vi "Initialise 3 cameras.vi"() -> (0 "Error Out":errorcluster, 1 "Blue camera ref":refnum<k24>, 2 "Green camera ref":refnum<k24>, 3 "Red camera ref":refnum<k24>)   [LabVIEW 2017]
uses:
  C:/Program Files/National Instruments/LabVIEW 2017/instr.lib/IDS/ueye.NET/uEyeDotNet.dll
panel:
  out "Serial Number 3":string
  out "Serial Number 2":string
  out "Serial Number 1":string
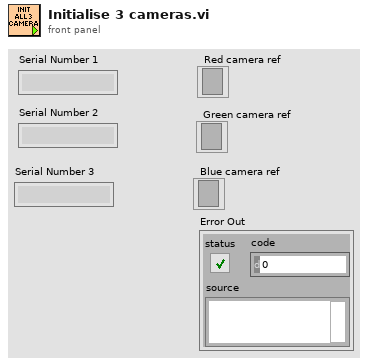
[diagram p1: front panel]
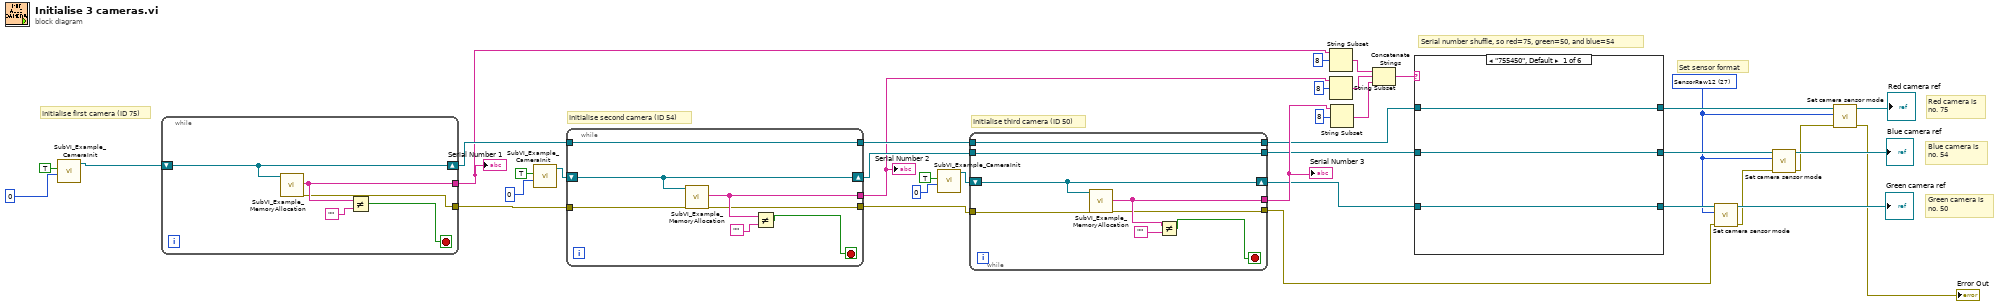
[diagram p0: block diagram]
diagram:
  w1 = 27 items=["BGRA8Packed"=0, "BGR8Packed"=1, "BGR565Packed"=2, "BGR5Packed"=3, "Mono8"=6, "SensorRaw8"=11, "UYVYPacked"=12, "UYVYMonoPacked"=13, "UYVYBayerPacked"=14, "CBYCRYPacked"=23, "BGRY8Packed"=24, "BGR10Packed"=25, "Mono12"=26, "SensorRaw12"=27, "Mono16"=28, "SensorRaw16"=29, "BGR12Unpacked"=30, "BGRA12Unpacked"=31, "Jpeg"=32, "BGR10Unpacked"=35, "RGBA8Packed"=128, "RGB8Packed"=129, "RGBY8Packed"=152, "RGB10Packed"=153, "RGB12Unpacked"=158, "RGBA12Unpacked"=159, "RGB10Unpacked"=163, "RGB8Planar"=8321, "PreferPackedSourceFormat"=16384] ("mode")
  # "Set sensor format"
  # "Red camera is \nno. 75"
  # "Green camera is \nno. 50"
  # "Blue camera is \nno. 54"
  # "Serial number shuffle, so red=75, green=50, and blue=54"
  # "Initialise third camera (ID 50)"
  # "Initialise second camera (ID 54)"
  # "Initialise first camera (ID 75)"
  n1 = call <instrlib>:"SubVI_Example_CameraInit.vi"("Camera ID"=0, "Init Camera Flag"=TRUE) -> (".NET (Reference)"=w36:refnum<k24>)  [unwired: 8 in, 1 out]
  n2 = while {
    shift-right: [w43] -> w32
    shift-left: w36 -> [w43]
    tunnel: [w40] -> w26
    tunnel: [w39] -> w13
    stop <- w41 stop-if-true
    n3 = call <instrlib>:"SubVI_Example_MemoryAllocation.vi"(".NET (Reference)"=w43) -> ("Serial Number"=w40:string, "Error Out"=w39:errorcluster)  [unwired: 14 in, 3 out]
    n4 = Not Equal?(x=w40, y="") -> (x != y?=w41:bool)
  }
  "Serial Number 1" <- w26
  n5 = call <instrlib>:"SubVI_Example_CameraInit.vi"("Camera ID"=0, "Init Camera Flag"=TRUE) -> (".NET (Reference)"=w35:refnum<k24>)  [unwired: 8 in, 1 out]
  n6 = while {
    shift-right: [w50] -> w27
    shift-left: w35 -> [w50]
    tunnel: [w47] -> w22
    tunnel: w32 -> [w46]
    tunnel: [w46] -> w28
    tunnel: w13 -> [w45]
    tunnel: [w44] -> w12
    stop <- w48 stop-if-true
    n7 = call <instrlib>:"SubVI_Example_MemoryAllocation.vi"(".NET (Reference)"=w50, "Error In"=w45) -> ("Serial Number"=w47:string, "Error Out"=w44:errorcluster)  [unwired: 13 in, 3 out]
    n8 = Not Equal?(x=w47, y="") -> (x != y?=w48:bool)
  }
  "Serial Number 2" <- w22
  n9 = call <instrlib>:"SubVI_Example_CameraInit.vi"("Camera ID"=0, "Init Camera Flag"=TRUE) -> (".NET (Reference)"=w29:refnum<k24>)  [unwired: 8 in, 1 out]
  n10 = while {
    shift-right: [w58] -> w14
    shift-left: w29 -> [w58]
    tunnel: [w55] -> w21
    tunnel: w28 -> [w53]
    tunnel: w27 -> [w54]
    tunnel: [w54] -> w15
    tunnel: [w53] -> w16
    tunnel: w12 -> [w52]
    tunnel: [w51] -> w5
    stop <- w56 stop-if-true
    n11 = call <instrlib>:"SubVI_Example_MemoryAllocation.vi"(".NET (Reference)"=w58, "Error In"=w52) -> ("Serial Number"=w55:string, "Error Out"=w51:errorcluster)  [unwired: 13 in, 3 out]
    n12 = Not Equal?(x=w55, y="") -> (x != y?=w56:bool)
  }
  "Serial Number 3" <- w21
  n13 = String Subset(string=w26, offset (0)=8) -> (substring=w20:string)  [unwired: 1 in]
  n14 = String Subset(string=w22, offset (0)=8) -> (substring=w19:string)  [unwired: 1 in]
  n15 = String Subset(string=w21, offset (0)=8) -> (substring=w18:string)  [unwired: 1 in]
  n16 = Concatenate Strings(w20, w19, w18) -> (w17:string)
  n17 = case shown="\"755450\", Default" w17 {
    tunnel: w16 -> [w61 w64 w67 w70 w73 w76]
    tunnel: w15 -> [w60 w63 w66 w69 w72 w75]
    tunnel: w14 -> [w59 w62 w65 w68 w71 w74]
    tunnel: [w61 w64 w66 w68 w72 w74] -> w11
    tunnel: [w60 w62 w67 w70 w71 w75] -> w9
    tunnel: [w59 w63 w65 w69 w73 w76] -> w7
    frame "755450", Default {
    }
    frame "755054" {
    }
    frame "547550" {
    }
    frame "545075" {
    }
    frame "507554" {
    }
    frame "505475" {
    }
  }
  n18 = call "Set camera sensor mode.vi"("Error In"=w5, "mode"=w1, "Camera reference in"=w7) -> ("Error Out"=w4:errorcluster, "Camera reference out"=→"Green camera ref":refnum<k24>)  [unwired: 6 in]
  n19 = call "Set camera sensor mode.vi"("Error In"=w4, "mode"=w1, "Camera reference in"=w9) -> ("Error Out"=w3:errorcluster, "Camera reference out"=→"Blue camera ref":refnum<k24>)  [unwired: 6 in]
  n20 = call "Set camera sensor mode.vi"("Error In"=w3, "mode"=w1, "Camera reference in"=w11) -> ("Error Out"=→"Error Out":errorcluster, "Camera reference out"=→"Red camera ref":refnum<k24>)  [unwired: 6 in]
